vi "InterComm.vi"(10 "intercomm configuration":T1) -> (0 "last error":errorcluster)   [LabVIEW 2018]
uses:
  Custom/S4msg.ctl
  <vilib>/LabVIEW Open Source Project/MQTT Client/Client class/Client.lvclass/Client.ctl
  <vilib>/LabVIEW Open Source Project/MQTT Connection/MQTT_Base/Base Class/MQTT_Base.lvclass/MQTT_Base.ctl
  <vilib>/addons/zeromq/socket_type.ctl
  <vilib>/LabVIEW Open Source Project/Connection/Connection.TCP/Connection.TCP.lvclass
  C:/Program Files (x86)/National Instruments/LabVIEW 2018/vi.lib/LabVIEW Open Source Project/Connection/Connection/Connection.lvclass
  <vilib>/LabVIEW Open Source Project/MQTT Client/Client class/Client.lvclass
  C:/Program Files (x86)/National Instruments/LabVIEW 2018/vi.lib/LabVIEW Open Source Project/MQTT Connection/MQTT_Base/Base Class/MQTT_Base.lvclass
  <vilib>/LabVIEW Open Source Project/MQTT Control Packets/Control Packets/PUBLISH/PUBLISH.lvclass
  <vilib>/LabVIEW Open Source Project/MQTT Connection/MQTT_Base/Base Class/MQTT_Base.lvclass
  <vilib>/LabVIEW Open Source Project/Connection/Connection.LocalQueue/Connection.LocalQueue.lvclass
  <vilib>/addons/zeromq/zeromq.lvlib
  <vilib>/addons/zeromq/zmq_context.lvclass
  <vilib>/addons/zeromq/zmq_socket.lvclass
panel:
  in  "port":u16=54165
  in  "address":string="localhost"
  out "S4ICS_status":string caption="Status received from S4ICS"
  out "S4ICS_command":string caption="Command sent to S4ICS"
  in  "Stop Client":bool
  out "channel":T2(tab)
  in  "Status":bool
  in  "ExecuteCmd":bool
  in  "command":string(combo)="S4ICS" caption="Available S4ICS Commands"
  in  "ms send message":i32=2000
  in  "ms rec message":i32=2000
  in  "ms create listener":i32=2000
  in  "listen timeout":i32=50 caption="Listenning timeout"
  out "local IP 2":string
  out "local IP 1":string
  in  "connection ID":refnum<k5>
  in  "Connection":bool
  out "Published":bool
  in  "S4ICS Status Topic":string="SPARC4 STATUS" caption="Publishing S4ICS Status Topic Name"
  in  "S4ICS Cmd Topic":string="SPARC4 COMMAND" caption="Subscribing S4ICS Command Topic Name"
  in  "Command Subscribe":bool
  out "Unsuback":bool
  out "Suback":bool
  # "S4ICS INTERCOMM"
  # "COMMUNICATION CHANNEL"
  # "TIMEOUT"
  # "LOCAL NETWORK CARDS"
  # "address\ntcp://127.0.0.1"
  # "port\n5555"
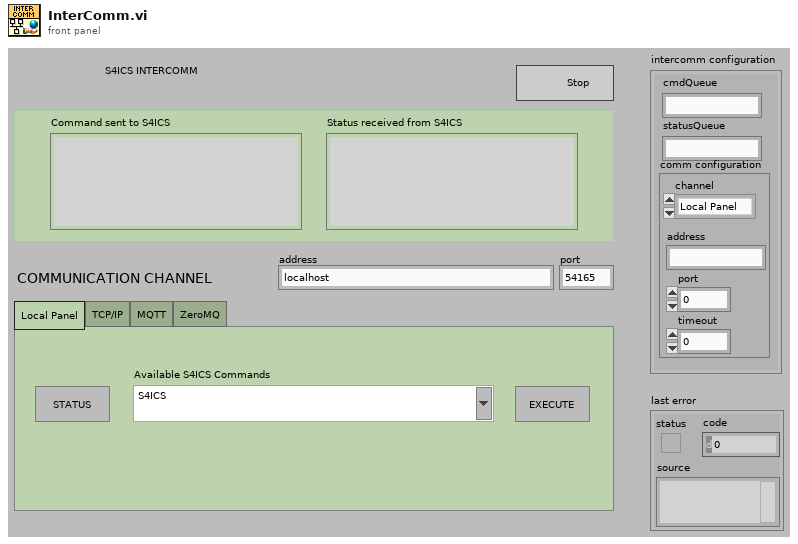
[diagram p1: front panel]
types:
  T1 = cluster{"S4commandQueueName":string, "S4statusQueueName":string, "comm configuration":cluster{"channel":enum32{"Local Panel", "Inner TCP/IP", "Outer TCP/IP", "MQTT", "ZeroMQ"}, "address":string, "port":u16, "timeout":i32}}
  T2 = enum32{"Local Panel", "TCP/IP", "MQTT", "ZeroMQ"}
  T3 = typedef "S4msg.ctl" = cluster{"msg topic":string, "msg data":variant}
  T4 = cluster{"channel":enum32{"Local Panel", "Inner TCP/IP", "Outer TCP/IP", "MQTT", "ZeroMQ"}, "address":string, "port":u16, "timeout":i32}
  T5 = enum32{"Local Panel", "Inner TCP/IP", "Outer TCP/IP", "MQTT", "ZeroMQ"}
  T6 = enum16{"Standard", "Buffered", "CRLF", "Immediate"}
  T7 = typedef "zeromq.lvlib/socket_type.ctl" = enum8{"ZMQ_PAIR", "ZMQ_PUB", "ZMQ_SUB", "ZMQ_REQ", "ZMQ_REP", "ZMQ_DEALER", "ZMQ_ROUTER", "ZMQ_PULL", "ZMQ_PUSH", "ZMQ_XPUB", "ZMQ_XSUB", "ZMQ_STREAM", "ZMQ_SERVER", "ZMQ_CLIENT", "ZMQ_RADIO", "ZMQ_DISH", "ZMQ_GATHER", "ZMQ_SCATTER", "ZMQ_DGRAM"}
  T8 = typedef "MQTT Client.lvlib/Client.lvclass/Public Events -- cluster.ctl" = cluster{"Connection Status":refnum<user-event>, "Connected":refnum<user-event>, "Application Message":refnum<user-event>}
  T9 = typedef "MQTT Base.lvlib/MQTT_Base.lvclass/Public Events -- cluster.ctl" = cluster{"Stop Event":refnum<user-event>, "Error Event":refnum<user-event>, "Inbound Message":refnum<user-event>}
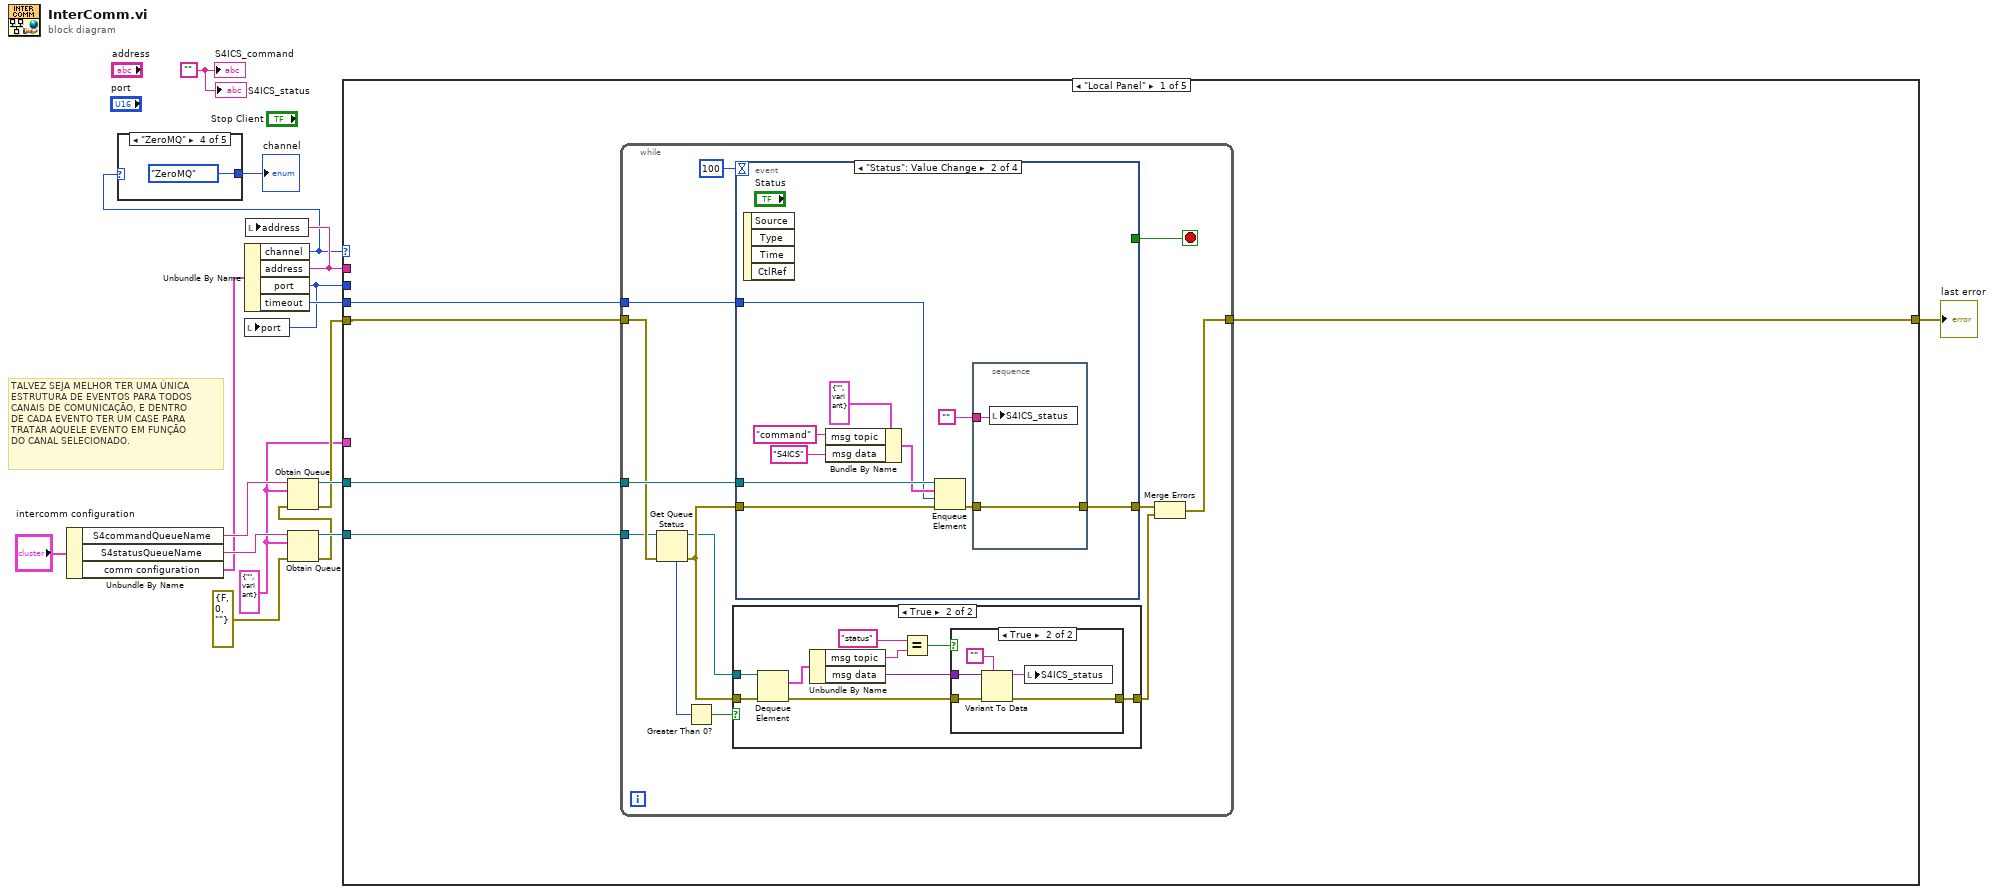
[diagram p0: block diagram]
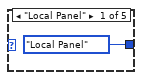
[diagram p2: hidden frame]
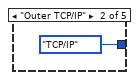
[diagram p3: hidden frame]
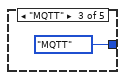
[diagram p4: hidden frame]
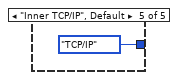
[diagram p5: hidden frame]
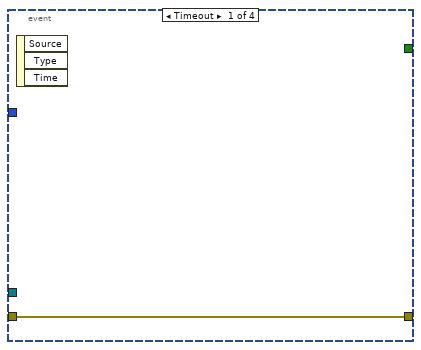
[diagram p8: hidden frame]
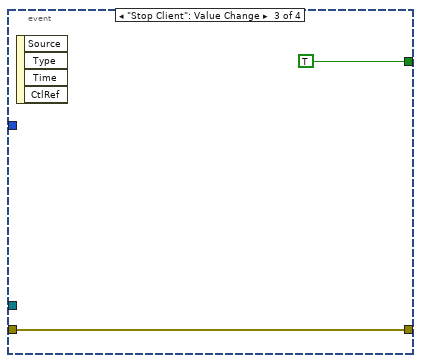
[diagram p9: hidden frame]
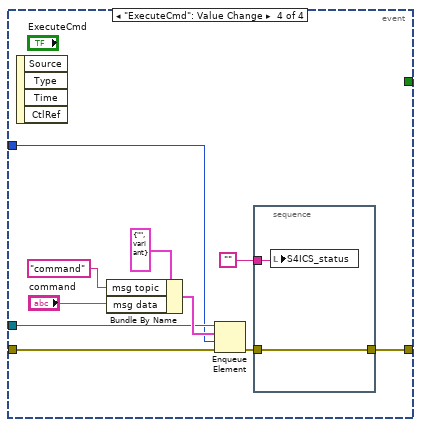
[diagram p10: hidden frame]
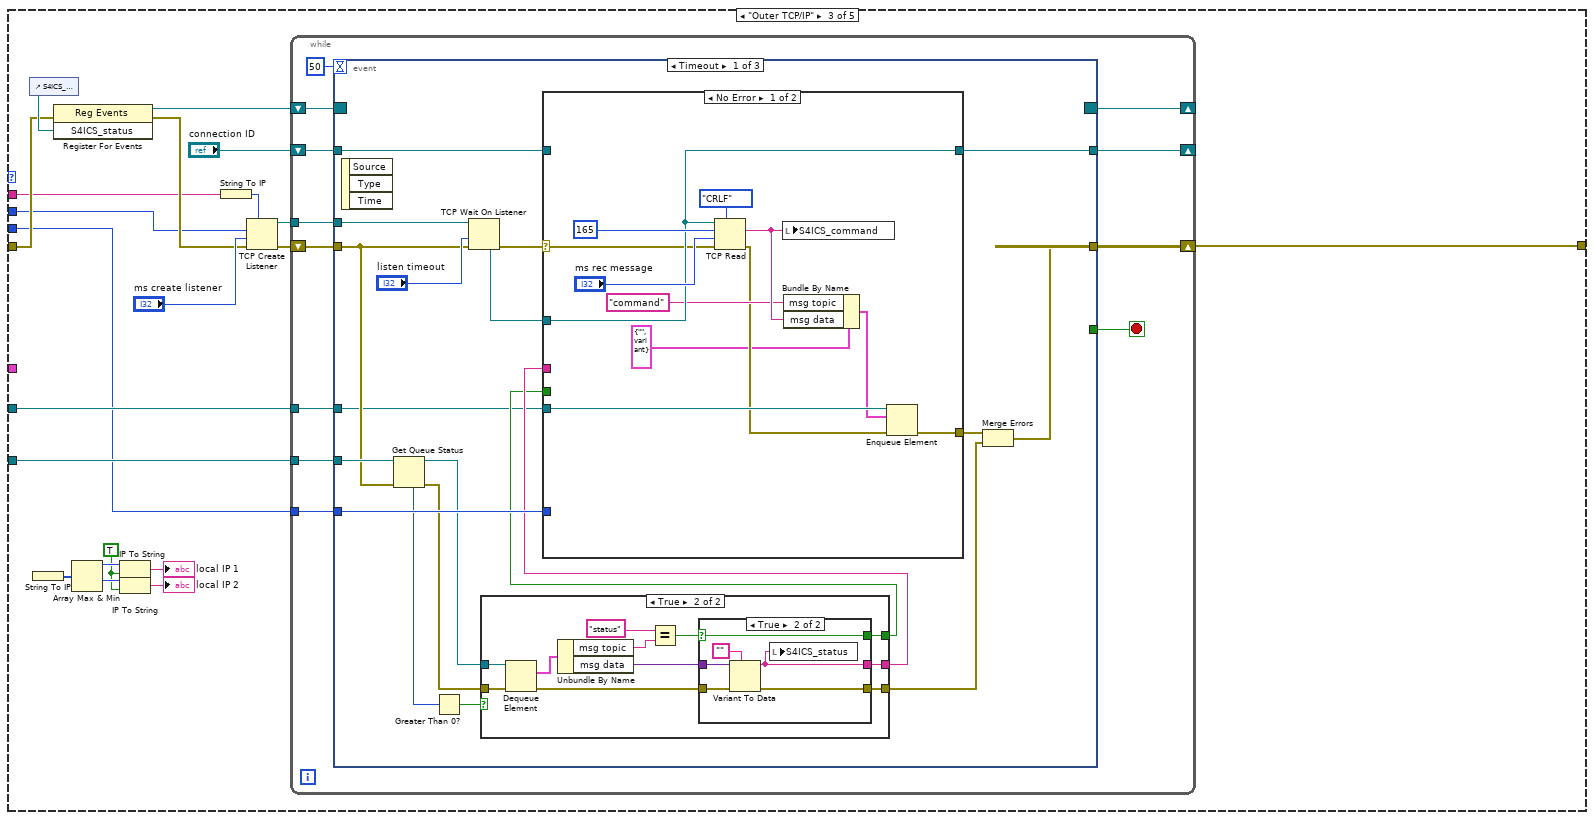
[diagram p12: hidden frame]
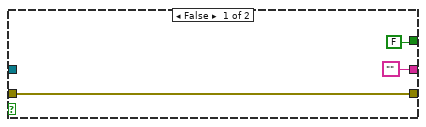
[diagram p13: hidden frame]
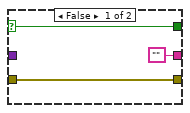
[diagram p14: hidden frame]
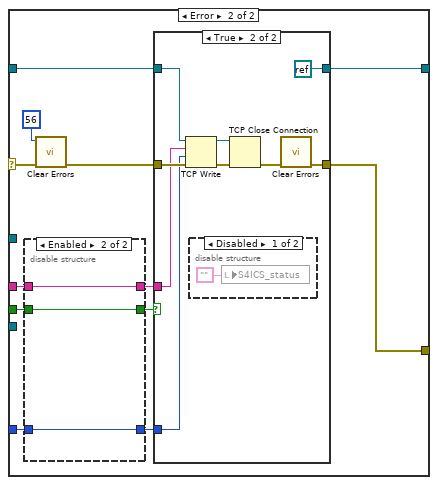
[diagram p15: hidden frame]
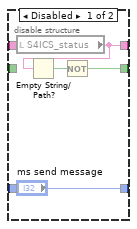
[diagram p16: hidden frame]
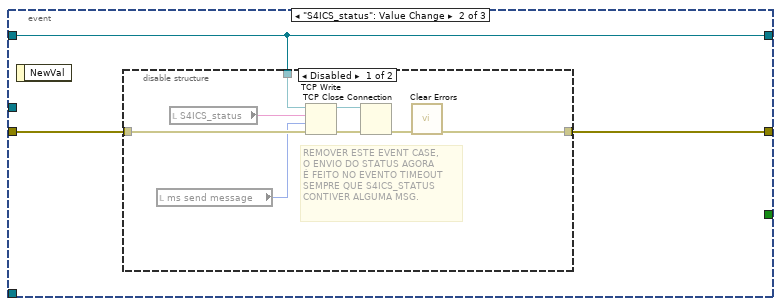
[diagram p19: hidden frame]
diagram:
  w1 = T3 {"msg topic"="", "msg data"=variant} ("S4msg")
  w16 = ""
  # "TALVEZ SEJA MELHOR TER UMA ÚNICA\nESTRUTURA DE EVENTOS PARA TODOS\nCANAIS DE COMUNICAÇÃO, E DENTRO\nDE CADA EVENTO TER UM CASE PARA\nTRATAR AQUELE EVENTO EM FUNÇÃO\nDO CANAL SELECIONADO."
  n1 = Unbundle By Name("intercomm configuration") -> ("S4commandQueueName"=w13:string, "S4statusQueueName"=w14:string, "comm configuration"=w6:T4)
  n2 = Unbundle By Name(w6) -> ("channel"=w2:T5, "address"=w4:string, "port"=w3:u16, "timeout"=w5:i32)
  n3 = case shown="\"ZeroMQ\"" w2 {
    tunnel: [T2."Local Panel" ("channel") T2."TCP/IP" ("channel") T2."MQTT" ("channel") T2."ZeroMQ" ("channel") T2."TCP/IP" ("channel")] -> w7
    frame "Local Panel" {
    }
    frame "Outer TCP/IP" {
    }
    frame "MQTT" {
    }
    frame "ZeroMQ" {
    }
    frame "Inner TCP/IP", Default {
    }
  }
  "channel" <- w7
  n4 = local write "port"(w3) -> ()
  n5 = local write "address"(w4) -> ()
  n6 = Obtain Queue(name (unnamed)=w14, element data type=w1, error in (no error)=errorcluster {"status"=FALSE, "code"=0, "source"=""}) -> (queue out=w11:refnum<queue>, error out=w8:errorcluster)  [unwired: 2 in, 1 out]
  n7 = Obtain Queue(name (unnamed)=w13, element data type=w1, error in (no error)=w8) -> (queue out=w12:refnum<queue>, error out=w10:errorcluster)  [unwired: 2 in, 1 out]
  n8 = case shown="\"Local Panel\"" w2 {
    tunnel: [w25 w84 w95 w251 w450] -> w17
    tunnel: w10 -> [w27 w84 w93 w250 w451]
    tunnel: w12 -> [w26 _ w88 w221 w449]
    tunnel: w11 -> [w24 _ w89 w220 w448]
    tunnel: w4 -> [_ _ w87 w224 w440]
    tunnel: w3 -> [_ _ w86 w223 w441]
    tunnel: w5 -> [w23 _ w85 w222 w442]
    tunnel: w1 -> [_ _ _ _ w439]
    frame "Local Panel" {
      n9 = while {
        tunnel: w27 -> [w37]
        tunnel: w26 -> [w38]
        tunnel: [w30] -> w25
        tunnel: w24 -> [w36]
        tunnel: w23 -> [w28]
        stop <- w39 stop-if-true
        n10 = Get Queue Status(queue=w36, error in (no error)=w37) -> (queue out=w32:refnum<queue>, error out=w33:errorcluster, # elements in queue=w35:i32)  [unwired: 1 in, 5 out]
        n11 = Greater Than 0?(x=w35) -> (x > 0?=w34:bool)
        n12 = case shown="True" w34 {
          tunnel: w33 -> [w41 w50]
          tunnel: w32 -> [_ w49]
          tunnel: [w41 w42] -> w29
          frame False {
          }
          frame True {
            n13 = Dequeue Element(queue=w49, error in (no error)=w50) -> (element=w48:T3, error out=w43:errorcluster)  [unwired: 1 in, 2 out]
            n14 = Unbundle By Name(w48) -> ("msg topic"=w46:string, "msg data"=w44:variant)
            n15 = Equal?(x="status" ("msg topic"), y=w46) -> (x = y?=w47:bool)
            n16 = case shown="True" w47 {
              tunnel: w44 -> [_ w56]
              tunnel: w43 -> [w51 w55]
              tunnel: [w51 w54] -> w42
              frame False {
              }
              frame True {
                n17 = Variant To Data(error in=w55, type="", Variant=w56) -> (data=w52:string, error out=w54:errorcluster)
                n18 = local write "S4ICS_status"(w52) -> ()
              }
            }
          }
        }
        n19 = event shown="[1] \"Status\": Value Change" {
          selector: _ -> [_ _ _ _]
          dyn-events: _ -> [_ _ _ _]
          timeout: 100 -> [_ _ _ _]
          tunnel: [_ _ TRUE _] -> w39
          tunnel: w38 -> [_ w67 _ w78]
          tunnel: [w57 w65 w70 w76] -> w31
          tunnel: w33 -> [w57 w62 w70 w77]
          tunnel: w28 -> [_ w59 _ w73]
          event Timeout {
            n20 = event-data() -> ()  [unwired: 1 in, 3 out]
          }
          event "Status": Value Change {
            n21 = event-data() -> ()  [unwired: 1 in, 4 out]
            n22 = Bundle By Name(cluster=T3 {"msg topic"="", "msg data"=variant} ("S4msg"), "msg topic"="command", "msg data"="S4ICS") -> (w66:T3)
            n23 = Enqueue Element(queue=w67, element=w66, timeout in ms (-1)=w59, error in (no error)=w62) -> (error out=w64:errorcluster)  [unwired: 2 out]
            n24 = stacked-sequence {
              tunnel: [w69] -> w65
              tunnel: w64 -> [w69]
              tunnel: "" -> [w68]
              frame #0 {
                n25 = local write "S4ICS_status"(w68) -> ()
              }
            }
          }
          event "Stop Client": Value Change {
            n26 = event-data() -> ()  [unwired: 1 in, 4 out]
          }
          event "ExecuteCmd": Value Change {
            n27 = event-data() -> ()  [unwired: 1 in, 4 out]
            n28 = Bundle By Name(cluster=T3 {"msg topic"="", "msg data"=variant} ("S4msg"), "msg topic"="command", "msg data"="command") -> (w81:T3)
            n29 = Enqueue Element(queue=w78, element=w81, timeout in ms (-1)=w73, error in (no error)=w77) -> (error out=w80:errorcluster)  [unwired: 2 out]
            n30 = stacked-sequence {
              tunnel: [w83] -> w76
              tunnel: w80 -> [w83]
              tunnel: "" -> [w82]
              frame #0 {
                n31 = local write "S4ICS_status"(w82) -> ()
              }
            }
          }
        }
        n32 = Merge Errors(w31, w29) -> (w30:errorcluster)
      }
    }
    frame "Inner TCP/IP", Default {
    }
    frame "Outer TCP/IP" {
      w102 = TRUE
      n33 = control-ref of="S4ICS_status"() -> (w94:refnum<vi>)
      n34 = String To IP() -> (0:w105:u32[])  [unwired: 1 in]
      n35 = register-events(error in=w93, w94) -> (reference out=w91:refnum<event-registration>, error out=w92:errorcluster)  [unwired: 1 in]
      n36 = Array Max & Min(array=w105) -> (max value=w104:u32, min value=w103:u32)  [unwired: 2 out]
      n37 = IP To String(1:w102, 2:w104) -> (0:→"local IP 1":string)
      n38 = IP To String(1:w102, 2:w103) -> (0:→"local IP 2":string)
      n39 = String To IP(1:w87) -> (0:w99:u32)
      n40 = TCP Create Listener(7:w99, 8:w92, 9:"ms create listener", 10:w86) -> (0:w98:errorcluster, 3:w97:refnum<k5>)  [unwired: 1 in, 1 out]
      n41 = while {
        tunnel: w97 -> [w116]
        shift-right: [w113] -> w95
        shift-left: w98 -> [w117]
        shift-right: [w110] -> _
        shift-left: "connection ID" -> [w111]
        shift-right: [w109] -> _
        shift-left: w91 -> [w112]
        tunnel: w89 -> [w108]
        tunnel: w88 -> [w107]
        tunnel: w85 -> [w106]
        stop <- w114 stop-if-true
        n42 = event shown="[0] Timeout" {
          selector: w112 -> [_ _ _]
          dyn-events: [_ _ _] -> w109
          timeout: 50 -> [_ _ _]
          tunnel: w117 -> [w125 w205 w219]
          tunnel: w116 -> [w136 _ w218]
          tunnel: [_ _ TRUE] -> w114
          tunnel: [w118 w204 w216] -> w113
          tunnel: w111 -> [w131 w203 w215]
          tunnel: [w132 w203 w215] -> w110
          tunnel: w106 -> [w130 _ _]
          tunnel: w108 -> [w129 _ _]
          tunnel: w107 -> [w121 _ _]
          event Timeout {
            n43 = event-data() -> ()  [unwired: 1 in, 3 out]
            n44 = Get Queue Status(queue=w129, error in (no error)=w125) -> (queue out=w124:refnum<queue>, error out=w126:errorcluster, # elements in queue=w128:i32)  [unwired: 1 in, 5 out]
            n45 = Greater Than 0?(x=w128) -> (x > 0?=w127:bool)
            n46 = TCP Wait On Listener(8:w125, 9:"listen timeout", 11:w136) -> (0:w134:errorcluster, 4:w133:refnum<k5>)  [unwired: 1 in, 3 out]
            n47 = case shown="True" w127 {
              tunnel: w126 -> [w139 w150]
              tunnel: w124 -> [_ w149]
              tunnel: [w139 w142] -> w119
              tunnel: ["" w141] -> w123
              tunnel: [FALSE w140] -> w122
              frame False {
              }
              frame True {
                n48 = Dequeue Element(queue=w149, error in (no error)=w150) -> (element=w148:T3, error out=w143:errorcluster)  [unwired: 1 in, 2 out]
                n49 = Unbundle By Name(w148) -> ("msg topic"=w146:string, "msg data"=w144:variant)
                n50 = Equal?(x="status" ("msg topic"), y=w146) -> (x = y?=w147:bool)
                n51 = case shown="True" w147 {
                  selector: w147 -> [w151 w154]
                  tunnel: w144 -> [_ w159]
                  tunnel: w143 -> [w153 w158]
                  tunnel: [w153 w157] -> w142
                  tunnel: ["" w155] -> w141
                  tunnel: [w151 w154] -> w140
                  frame False {
                  }
                  frame True {
                    n52 = Variant To Data(error in=w158, type="", Variant=w159) -> (data=w155:string, error out=w157:errorcluster)
                    n53 = local write "S4ICS_status"(w155) -> ()
                  }
                }
              }
            }
            n54 = case shown="No Error" w134 {
              selector: w134 -> [w166 w183]
              tunnel: w133 -> [w168 _]
              tunnel: [w161 w180] -> w120
              tunnel: [w168 w178] -> w132
              tunnel: w131 -> [_ w179]
              tunnel: w123 -> [_ w173]
              tunnel: w130 -> [_ w176]
              tunnel: w122 -> [_ w172]
              tunnel: w121 -> [w167 _]
              frame No Error {
                n55 = TCP Read(connection ID=w168, bytes to read=165, error in (no error)=w166, 7:T6."CRLF" ("mode (standard)"), 9:"ms rec message") -> (data out=w165:string, error out=w162:errorcluster)  [unwired: 1 out]
                n56 = local write "S4ICS_command"(w165) -> ()
                n57 = Bundle By Name(cluster=T3 {"msg topic"="", "msg data"=variant} ("S4msg"), "msg topic"="command", "msg data"=w165) -> (w163:T3)
                n58 = Enqueue Element(queue=w167, element=w163, error in (no error)=w162) -> (error out=w161:errorcluster)  [unwired: 1 in, 2 out]
              }
              frame Error {
                n59 = disable-structure shown="Enabled" {
                  disable-tunnel: ["ms send message" w190] -> w177
                  disable-tunnel: w176 -> [_ w190]
                  disable-tunnel: [w184 w189] -> w175
                  disable-tunnel: [w185 w188] -> w174
                  disable-tunnel: w173 -> [_ w189]
                  disable-tunnel: w172 -> [_ w188]
                  frame Disabled {
                    n60 = local read "S4ICS_status"() -> (w184:string)
                    n61 = Empty String/Path?(string/path=w184) -> (empty?=w186:bool)
                    n62 = Not(x=w186) -> (.not. x?=w185:bool)
                  }
                  frame Enabled {
                  }
                }
                n63 = call <vilib>:"Clear Errors.vi"("error in (no error)"=w183, "specific error code to clear (0: all)"=56) -> ("error out"=w181:errorcluster)  [unwired: 4 in, 1 out]
                n64 = case shown="True" w174 {
                  tunnel: w181 -> [w192 w198]
                  tunnel: [w192 w197] -> w180
                  tunnel: w179 -> [w191 w196]
                  tunnel: [w191 refnum<k0> refnum] -> w178
                  tunnel: w175 -> [_ w195]
                  tunnel: w177 -> [_ w193]
                  frame False {
                  }
                  frame True {
                    n65 = TCP Write(connection ID=w196, data in=w195, error in (no error)=w198, 9:w193) -> (connection ID out=w199:refnum<k5>, error out=w200:errorcluster)  [unwired: 1 out]
                    n66 = disable-structure shown="Disabled" {
                      frame Disabled {
                        n67 = local write "S4ICS_status"("") -> ()
                      }
                      frame Enabled {
                      }
                    }
                    n68 = TCP Close Connection(connection ID=w199, error in (no error)=w200) -> (error out=w201:errorcluster)  [unwired: 1 in, 1 out]
                    n69 = call <vilib>:"Clear Errors.vi"("error in (no error)"=w201) -> ("error out"=w197:errorcluster)  [unwired: 5 in, 1 out]
                  }
                }
              }
            }
            n70 = Merge Errors(w120, w119) -> (w118:errorcluster)
          }
          event "S4ICS_status": Value Change {
            n71 = event-data() -> ()  [unwired: 1 in, 1 out]
            n72 = disable-structure shown="Disabled" {
              disable-tunnel: w205 -> [w213 w214]
              disable-tunnel: [w210 w214] -> w204
              disable-tunnel: w203 -> [w208 _]
              frame Disabled {
                # "REMOVER ESTE EVENT CASE,\nO ENVIO DO STATUS AGORA\nÉ FEITO NO EVENTO TIMEOUT\nSEMPRE QUE S4ICS_STATUS\nCONTIVER ALGUMA MSG."
                n73 = local read "ms send message"() -> (w206:i32)
                n74 = local read "S4ICS_status"() -> (w207:string)
                n75 = TCP Write(connection ID=w208, data in=w207, error in (no error)=w213, 9:w206) -> (connection ID out=w209:refnum<k5>, error out=w211:errorcluster)  [unwired: 1 out]
                n76 = TCP Close Connection(connection ID=w209, error in (no error)=w211) -> (error out=w212:errorcluster)  [unwired: 1 in, 1 out]
                n77 = call <vilib>:"Clear Errors.vi"("error in (no error)"=w212) -> ("error out"=w210:errorcluster)  [unwired: 5 in, 1 out]
              }
              frame Enabled {
              }
            }
          }
          event "Stop Client": Value Change {
            n78 = event-data() -> ()  [unwired: 1 in, 3 out]
            n79 = TCP Close Connection(connection ID=w218, error in (no error)=w219) -> (error out=w216:errorcluster)  [unwired: 1 in, 1 out]
          }
        }
      }
    }
    frame "MQTT" {
      w225 = FALSE
      # "QUANDO O VI RODAR,\nACIONAR  CONNECTION E\nSUBSCRIBE AUTOMATICAMENTE"
      n80 = disable-structure shown="Enabled" {
        disable-tunnel: [_ w267] -> w232
        disable-tunnel: [_ w266] -> w231
        disable-tunnel: w250 -> [_ w265]
        disable-tunnel: w224 -> [_ w264]
        disable-tunnel: w223 -> [_ w263]
        frame Disabled {
          n81 = call <vilib>:"Configure Queue Connection.vi"("Queue Name"="queueName") -> ()  [unwired: 9 in, 2 out]
        }
        frame Enabled {
          n82 = call <vilib>:"Configure TCP Connection.vi"("error in (no error)"=w265, "remote port (80)"=w263, "address (localhost)"=w264) -> ("error out"=w266:errorcluster, "Connection.TCP"=w267:refnum<class "Connection.TCP.lvclass">)  [unwired: 7 in]
        }
      }
      n83 = call <vilib>:"Create MQTT Client.vi"("error in (no error)"=w231, "Connection Configuration"=w232) -> ("error out"=w235:errorcluster, "Client out"=w233:refnum<class "Client.lvclass">)  [unwired: 8 in]
      n84 = call <vilib>:"Read Public Events.vi"("error in (no error)"=w235, "Client in"=w233) -> ("error out"=w236:errorcluster, "Client Public Events"=w238:T8, "Client out"=w234:refnum<class "Client.lvclass">)  [unwired: 7 in]
      n85 = call <vilib>:"Read MQTT Public Events.vi"("error in (no error)"=w236, "MQTT_Base in"=w234) -> ("error out"=w237:errorcluster, "MQTT Public Events"=w245:T9, "MQTT_Base out"=w240:refnum<class "Client.lvclass">)  [unwired: 7 in]
      n86 = Unbundle By Name(w245) -> ("Stop Event"=w243:refnum<user-event>, "Error Event"=w244:refnum<user-event>)
      n87 = local write "Command Subscribe"(w225) -> ()
      n88 = local write "Connection"(w225) -> ()
      n89 = local write "Published"(w225) -> ()
      n90 = local write "Unsuback"(w225) -> ()
      n91 = local write "Suback"(w225) -> ()
      n92 = register-events(error in=w237, w243, w244, w238) -> (reference out=w241:refnum<event-registration>, error out=w239:errorcluster)  [unwired: 1 in]
      n93 = call <vilib>:"Start.vi"("error in (no error)"=w239, "MQTT_Base in"=w240) -> ("error out"=w229:errorcluster, "MQTT_Base out"=w228:refnum<class "Client.lvclass">)  [unwired: 7 in, 1 out]
      n94 = First Call?() -> (First Call?: T/F=w230:bool)
      n95 = case shown="True" w230 {
        tunnel: w229 -> [w252 w261]
        tunnel: w228 -> [w253 w260]
        tunnel: [w253 w258] -> w227
        tunnel: [w252 w256] -> w226
        frame False {
        }
        frame True {
          n96 = local read "S4ICS Cmd Topic"() -> (w254:string)
          n97 = call <vilib>:"Connect to Server.vi"("error in (no error)"=w261, "Client in"=w260) -> ("error out"=w257:errorcluster, "Client out"=w259:refnum<class "Client.lvclass">)  [unwired: 6 in, 2 out]
          n98 = call <vilib>:"Subscribe (Scalar).vi"("error in (no error)"=w257, "Topic Filter"=w254, "Client in"=w259) -> ("error out"=w256:errorcluster, "Ack"=w255:bool, "Client out"=w258:refnum<class "Client.lvclass">)  [unwired: 6 in]
          n99 = local write "Suback"(w255) -> ()
        }
      }
      n100 = while {
        shift-right: [w276] -> w242
        shift-left: w241 -> [w277]
        shift-right: [w273] -> w247
        shift-left: w227 -> [w274]
        shift-right: [w275] -> w249
        shift-left: w226 -> [w271]
        tunnel: w222 -> [w270]
        tunnel: w221 -> [w269]
        tunnel: w220 -> [w268]
        stop <- w272 stop-if-true
        n101 = case shown="No Error" w271 {
          selector: w271 -> [w281 w431]
          tunnel: w277 -> [w288 w434]
          tunnel: [w287 w434] -> w276
          tunnel: [w286 w429] -> w275
          tunnel: w274 -> [w284 w430]
          tunnel: [w283 w433] -> w273
          tunnel: [w282 w428] -> w272
          tunnel: w270 -> [w280 _]
          tunnel: w269 -> [w279 _]
          tunnel: w268 -> [w278 _]
          frame No Error {
            n102 = event shown="[1] <Client Public Events.Application Message>: User Event" {
              selector: w288 -> [_ _ _ _ _ _ _]
              dyn-events: [_ _ _ _ _ _ _] -> w287
              timeout: 50 -> [_ _ _ _ _ _ _]
              tunnel: w281 -> [w294 w341 w377 w384 w410 w412 w425]
              tunnel: [w297 w344 w377 w380 w410 w413 w425] -> w286
              tunnel: [_ _ TRUE _ TRUE _ w427] -> w282
              tunnel: w284 -> [w296 w347 w375 w385 w411 w416 w426]
              tunnel: [w298 w346 w375 w379 w411 w414 w426] -> w283
              tunnel: w280 -> [w289 w342 _ _ _ _ _]
              tunnel: w279 -> [w290 w343 _ _ _ _ _]
              tunnel: w278 -> [w291 _ _ _ _ _ _]
              event Timeout {
                n103 = event-data() -> ()  [unwired: 1 in, 1 out]
                n104 = call <vilib>:"isConnected.vi"("error in (no error)"=w294, "Client in"=w296) -> ("error out"=w293:errorcluster, "connected"=w292:bool, "Client out"=w295:refnum<class "Client.lvclass">)  [unwired: 7 in]
                n105 = case shown="True" w292 {
                  tunnel: [w301 w309] -> w298
                  tunnel: [w300 w310] -> w297
                  tunnel: w295 -> [w301 w311]
                  tunnel: w293 -> [w300 w305]
                  tunnel: w291 -> [_ w306]
                  tunnel: w290 -> [_ _]
                  tunnel: w289 -> [_ w302]
                  frame False {
                    n106 = local write "Connection"(FALSE ("Connection")) -> ()
                  }
                  frame True {
                    n107 = Get Queue Status(queue=w306, error in (no error)=w305) -> (queue out=w303:refnum<queue>, error out=w304:errorcluster, # elements in queue=w308:i32)  [unwired: 1 in, 5 out]
                    n108 = Greater Than 0?(x=w308) -> (x > 0?=w307:bool)
                    n109 = case shown="True" w307 {
                      tunnel: w311 -> [w313 w325]
                      tunnel: [w312 w324] -> w310
                      tunnel: [w313 w323] -> w309
                      tunnel: w304 -> [w312 w316]
                      tunnel: w303 -> [_ w317]
                      tunnel: w302 -> [_ w314]
                      frame False {
                      }
                      frame True {
                        n110 = Dequeue Element(queue=w317, error in (no error)=w316) -> (element=w319:T3, error out=w322:errorcluster)  [unwired: 1 in, 2 out]
                        n111 = Unbundle By Name(w319) -> ("msg topic"=w320:string, "msg data"=w321:variant)
                        n112 = Equal?(x="status" ("msg topic"), y=w320) -> (x = y?=w315:bool)
                        n113 = case shown="True" w315 {
                          tunnel: w325 -> [w327 w339]
                          tunnel: [w326 w338] -> w324
                          tunnel: [w327 w337] -> w323
                          tunnel: w322 -> [w326 w333]
                          tunnel: w321 -> [_ w332]
                          tunnel: w314 -> [_ w328]
                          frame False {
                          }
                          frame True {
                            (unwired) "$events"
                            (unwired) "$SYS/#" ("Topic Name")
                            n114 = Variant To Data(error in=w333, type="", Variant=w332) -> (data=w329:string, error out=w330:errorcluster)
                            n115 = call <vilib>:"Publish.vi"("timeout (1000ms)"=w328, "error in (no error)"=w330, "Payload"=w329, "Topic Name (empty: Payload name)"="S4ICS Status Topic", "Client in"=w339) -> ("error out"=w338:errorcluster, "Published"=→"Published":bool, "Client out"=w337:refnum<class "Client.lvclass">)  [unwired: 4 in]
                            n116 = local write "S4ICS_status"("") -> ()
                          }
                        }
                      }
                    }
                  }
                }
              }
              event User Event {
                n117 = event-data() -> ("PUBLISH"=w349:refnum<class "PUBLISH.lvclass">)  [unwired: 1 in]
                n118 = call <vilib>:"getTopicName.vi"("error in (no error)"=w341, "PUBLISH in"=w349) -> ("error out"=w340:errorcluster, "Topic"=w345:string, "PUBLISH out"=w348:refnum<class "PUBLISH.lvclass">)  [unwired: 7 in]
                n119 = case shown="\"SPARC4 COMMAND\"" w345 {
                  tunnel: w348 -> [_ w362]
                  tunnel: w347 -> [w350 w365]
                  tunnel: w340 -> [w351 w364]
                  tunnel: [w350 w363] -> w346
                  tunnel: [w351 w352] -> w344
                  tunnel: w343 -> [_ w355]
                  tunnel: w342 -> [_ w354]
                  frame Default {
                  }
                  frame "SPARC4 COMMAND" {
                    n120 = call <vilib>:"Decode Application Message (Raw).vi"("error in (no error)"=w364, "PUBLISH"=w362, "Client in"=w365) -> ("error out"=w353:errorcluster, "Payload"=w361:u8[], "Client out"=w363:refnum<class "Client.lvclass">)  [unwired: 5 in, 1 out]
                    n121 = Byte Array To String(unsigned byte array=w361) -> (string=w360:string)
                    n122 = Match Pattern(string=w360, regular expression="S4ICS") -> (after substring=w357:string, offset past match=w358:i32)  [unwired: 1 in, 2 out]
                    n123 = Greater Than 0?(x=w358) -> (x > 0?=w356:bool)
                    n124 = case shown="True" w356 {
                      tunnel: w357 -> [_ w373]
                      tunnel: w355 -> [_ w374]
                      tunnel: w354 -> [_ w370]
                      tunnel: w353 -> [w366 w369]
                      tunnel: [w366 w368] -> w352
                      frame False {
                      }
                      frame True {
                        n125 = local write "S4ICS_command"(w373) -> ()
                        n126 = Bundle By Name(cluster=T3 {"msg topic"="", "msg data"=variant} ("S4msg"), "msg topic"="command", "msg data"=w373) -> (w371:T3)
                        n127 = Enqueue Element(queue=w374, element=w371, timeout in ms (-1)=w370, error in (no error)=w369) -> (error out=w368:errorcluster)  [unwired: 2 out]
                      }
                    }
                  }
                }
              }
              event User Event {
                n128 = event-data() -> ()  [unwired: 1 in, 1 out]
              }
              event "Command Subscribe": Value Change {
                n129 = event-data() -> ("NewVal"=w378:bool)  [unwired: 1 in]
                n130 = call <vilib>:"isConnected.vi"("error in (no error)"=w384, "Client in"=w385) -> ("error out"=w381:errorcluster, "connected"=w383:bool, "Client out"=w382:refnum<class "Client.lvclass">)  [unwired: 7 in]
                n131 = case shown="True" w383 {
                  tunnel: w382 -> [w386 w395]
                  tunnel: w381 -> [w387 w396]
                  tunnel: [w387 w391] -> w380
                  tunnel: [w386 w390] -> w379
                  tunnel: w378 -> [_ w389]
                  frame False {
                    n132 = local write "Connection"(FALSE ("Connection")) -> ()
                  }
                  frame True {
                    n133 = case shown="True" w389 {
                      tunnel: [w397 w405] -> w390
                      tunnel: [w398 w404] -> w391
                      tunnel: w395 -> [w402 w408]
                      tunnel: w396 -> [w401 w407]
                      tunnel: "S4ICS Cmd Topic" -> [w400 w406]
                      tunnel: [_ w403] -> w393
                      tunnel: [w399 _] -> w392
                      frame False {
                        n134 = call <vilib>:"Unsubscribe (Scalar).vi"("error in (no error)"=w401, "Topic Filter"=w400, "Client in"=w402) -> ("error out"=w398:errorcluster, "Ack"=w399:bool, "Client out"=w397:refnum<class "Client.lvclass">)  [unwired: 6 in]
                      }
                      frame True {
                        n135 = call <vilib>:"Subscribe (Scalar).vi"("error in (no error)"=w407, "Topic Filter"=w406, "Client in"=w408) -> ("error out"=w404:errorcluster, "Ack"=w403:bool, "Client out"=w405:refnum<class "Client.lvclass">)  [unwired: 6 in]
                      }
                    }
                    "Unsuback" <- w392
                    "Suback" <- w393
                  }
                }
              }
              event "Stop Client": Value Change {
                n136 = event-data() -> ()  [unwired: 1 in, 1 out]
              }
              event "Connection": Value Change {
                n137 = event-data() -> ("NewVal"=w415:bool)  [unwired: 1 in]
                n138 = case shown="True" w415 {
                  tunnel: w416 -> [w420 w424]
                  tunnel: [w419 w421] -> w414
                  tunnel: [w418 w422] -> w413
                  tunnel: w412 -> [w417 w423]
                  frame False {
                    n139 = call <vilib>:"Disconnect from Server.vi"("error in (no error)"=w417, "Client in"=w420) -> ("error out"=w418:errorcluster, "Client out"=w419:refnum<class "Client.lvclass">)  [unwired: 7 in, 1 out]
                  }
                  frame True {
                    n140 = call <vilib>:"Connect to Server.vi"("error in (no error)"=w423, "Client in"=w424) -> ("error out"=w422:errorcluster, "Client out"=w421:refnum<class "Client.lvclass">)  [unwired: 6 in, 2 out]
                  }
                }
              }
              event Panel Close? {
                w427 = TRUE
                n141 = event-data() -> ()  [unwired: 1 in, 4 out]
                n142 = event-data("Discard?"=w427) -> ()  [unwired: 1 in, 1 out]
              }
            }
          }
          frame Error {
            n143 = Unbundle By Name(w431) -> ("code"=w432:i32)
            n144 = local write "last error"(w431) -> ()
            n145 = case shown="Default" w432 {
              tunnel: w430 -> [w437 w438]
              tunnel: [w437 w438] -> w433
              tunnel: w431 -> [w436 _]
              tunnel: [w436 _] -> w429
              tunnel: [TRUE _] -> w428
              frame Default {
                # "Stop on Unhandled Error"
              }
              frame 56, 63, 66 {
                # "Disconnected"
              }
            }
          }
        }
      }
      n146 = call <vilib>:"Stop.vi"("error in (no error)"=w249, "MQTT_Base in"=w247) -> ("error out"=w248:errorcluster, "MQTT_Base out"=w246:refnum<class "Client.lvclass">)  [unwired: 7 in, 1 out]
      n147 = Unregister For Events(event registration refnum=w242) -> ()  [unwired: 1 in, 1 out]
      n148 = call <vilib>:"Destroy.vi"("error in (no error)"=w248, "MQTT_Base in"=w246) -> ("error out"=w251:errorcluster)  [unwired: 8 in, 1 out]
    }
    frame "ZeroMQ" {
      (unwired) "tcp://*:5555" ("endpoint")
      # "publisher command msg: @0ÿÿÿÿClient CommandS4ICS"
      # "Creates a reply (REP) socket and binds (listens to) address:port. Waits for a command message and puts it into \nS4commandQueue.  Waits againg for incoming data at S4statusQueue and replies it to the socket.\nThe receive call is blocking, and the example can be stopped by clicking Abort. Clean-up is done automatically."
      n149 = Number To Decimal String(number=w441) -> (decimal integer string=w446:string)  [unwired: 1 in]
      n150 = Concatenate Strings(w440, ":" ("endpoint"), w446) -> (w443:string)
      n151 = call <vilib>:"zmq_ctx_create.vi"("error in"=w451) -> ("error out"=w460:errorcluster, "context out"=w459:refnum<class "zmq_context.lvclass">)  [unwired: 3 in]
      n152 = call <vilib>:"zmq_socket.vi"("error in"=w460, "socket type"=socket_type."ZMQ_REP", "context in"=w459) -> ("error out"=w462:errorcluster, "socket out"=w461:refnum<class "zmq_socket.lvclass">, "context out"=w452:refnum<class "zmq_context.lvclass">)  [unwired: 2 in]
      n153 = Bundle By Name(cluster=w439, "msg topic"="command") -> (w444:T3)
      n154 = call <vilib>:"zmq_bind.vi"("error in"=w462, "endpoint"=w443, "socket in"=w461) -> ("error out"=w456:errorcluster, "socket out"=w457:refnum<class "zmq_socket.lvclass">)  [unwired: 1 in]
      n155 = while {
        tunnel: w457 -> [w476]
        tunnel: w456 -> [w477]
        tunnel: [w474] -> w455
        tunnel: [w473] -> w454
        tunnel: w449 -> [w472]
        tunnel: w448 -> [w470]
        tunnel: w442 -> [w471]
        tunnel: w444 -> [w463]
        stop <- w474 stop-if-true
        n156 = call <vilib>:"zmq_recv.vi"("error in"=w477, "socket in"=w476) -> ("error out"=w469:errorcluster, "data"=w466:string, "socket out"=w475:refnum<class "zmq_socket.lvclass">)  [unwired: 3 in, 2 out]
        n157 = local write "S4ICS_command"(w466) -> ()
        n158 = Bundle By Name(cluster=w463, "msg data"=w466) -> (w465:T3)
        n159 = Enqueue Element(queue=w472, element=w465, timeout in ms (-1)=w471, error in (no error)=w469) -> (error out=w464:errorcluster)  [unwired: 2 out]
        n160 = while {
          tunnel: w470 -> [w486]
          shift-right: [w480] -> w467
          shift-left: w464 -> [w485]
          tunnel: [w478] -> w468
          stop <- w479 stop-if-true
          n161 = Get Queue Status(queue=w486, error in (no error)=w485) -> (queue out=w483:refnum<queue>, error out=w482:errorcluster, # elements in queue=w484:i32)  [unwired: 1 in, 5 out]
          n162 = Greater Than 0?(x=w484) -> (x > 0?=w481:bool)
          n163 = case shown="True" w481 {
            tunnel: w482 -> [w488 w499]
            tunnel: w483 -> [_ w498]
            tunnel: [w488 w491] -> w480
            tunnel: [FALSE w490] -> w479
            tunnel: [_ w489] -> w478
            frame False {
            }
            frame True {
              n164 = Dequeue Element(queue=w498, error in (no error)=w499) -> (element=w497:T3, error out=w492:errorcluster)  [unwired: 1 in, 2 out]
              n165 = Unbundle By Name(w497) -> ("msg topic"=w495:string, "msg data"=w493:variant)
              n166 = Equal?(x="status" ("msg topic"), y=w495) -> (x = y?=w496:bool)
              n167 = case shown="True" w496 {
                selector: w496 -> [w500 w503]
                tunnel: w493 -> [_ w507]
                tunnel: w492 -> [w501 w506]
                tunnel: [w501 w505] -> w491
                tunnel: [w500 w503] -> w490
                tunnel: [_ w502] -> w489
                frame False {
                }
                frame True {
                  n168 = Variant To Data(error in=w506, type="", Variant=w507) -> (data=w502:string, error out=w505:errorcluster)
                }
              }
            }
          }
        }
        n169 = local write "S4ICS_status"(w468) -> ()
        n170 = call <vilib>:"zmq_send.vi"("error in"=w467, "data"=w468, "socket in"=w475) -> ("error out"=w474:errorcluster, "socket out"=w473:refnum<class "zmq_socket.lvclass">)  [unwired: 4 in]
      }
      n171 = call <vilib>:"zmq_close.vi"("error in"=w455, "socket"=w454) -> ("error out"=w453:errorcluster)  [unwired: 3 in]
      n172 = call <vilib>:"zmq_ctx_destroy.vi"("error in"=w453, "context in"=w452) -> ("error out"=w450:errorcluster)  [unwired: 3 in]
    }
  }
  "last error" <- w17
  "S4ICS_command" <- w16
  "S4ICS_status" <- w16
